vi "Database.Disconnect.vi"(8 "error in (no error)":errorcluster, 11 "Data in":T1) -> (0 "error out":errorcluster, 3 "Data out":T1)   [LabVIEW 2016]
doc: "Disconnect from database\n\nWabco 2017 All right reserved\nAuthor: maciej.szupienko@wabco-auto.com"
uses:
  Database.Data.ctl
  Database.Data.Sets.ctl
  Handler/Database.Handler.Data.Status.ctl
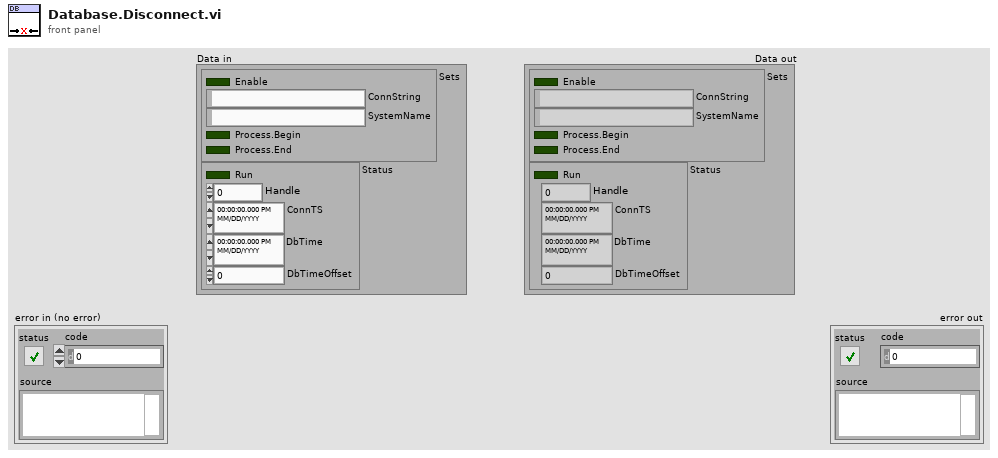
[diagram p1: front panel]
types:
  T1 = typedef "Database.Data.ctl" = cluster{"Sets":T2, "Status":T3}
  T2 = typedef "Database.Data.Sets.ctl" = cluster{"Enable":bool, "ConnString":string, "SystemName":string, "Process.Begin":bool, "Process.End":bool}
  T3 = typedef "Database.Handler.Data.Status.ctl" = cluster{"Run":bool, "Handle":i32, "ConnTS":timestamp, "DbTime":timestamp, "DbTimeOffset":dbl}
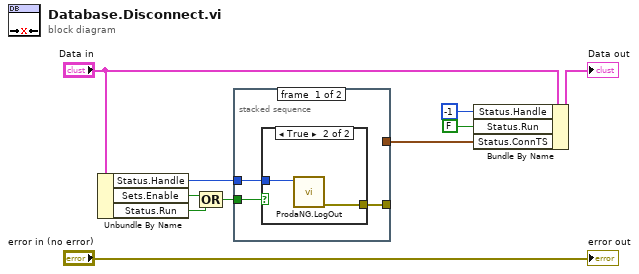
[diagram p0: block diagram]
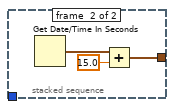
[diagram p3: hidden frame]
diagram:
  n1 = Unbundle By Name("Data in") -> ("Status.Handle"=w8:i32, "Sets.Enable"=w3:bool, "Status.Run"=w1:bool)
  n2 = Compound Arithmetic op=OR(w3, w1) -> (w2:bool)
  n3 = stacked-sequence {
    tunnel: w8 -> [w13 _]
    tunnel: [w12 _] -> _
    tunnel: [_ w16] -> w5
    tunnel: w2 -> [w11 _]
    frame #0 {
      n4 = case shown="True" w11 {
        tunnel: w13 -> [_ w15]
        tunnel: [_ w14] -> w12
        frame False {
        }
        frame True {
          n5 = call "ProdaNG.LogOut.vi"("dbHandleIn"=w15) -> ("error out"=w14:errorcluster)  [unwired: 10 in]
        }
      }
    }
    frame #1 {
      n6 = Get Date/Time In Seconds() -> (seconds since 1Jan1904=w18:timestamp)
      n7 = Add(x=w18, y=15.0) -> (x+y=w16:timestamp)
    }
  }
  n8 = Bundle By Name(cluster="Data in", "Status.Handle"=-1, "Status.Run"=FALSE ("Status.Connected"), "Status.ConnTS"=w5) -> (→"Data out":T1)
  "error out" <- "error in (no error)"
